vi "Get VIRef from ClassItem.vi"(8 "error in (no error)":errorcluster, 10 "Item Name":string, 11 "LVClassLibrary in":refnum<vi>) -> (0 "error out":errorcluster, 1 "Found ?":bool, 2 "VIref out":refnum<vi>, 3 "LVClassLibrary out":refnum<vi>)   [LabVIEW 2019, in "gRPC Scripting Tools.lvlib"]
uses:
  gRPC Scripting Tools.lvlib
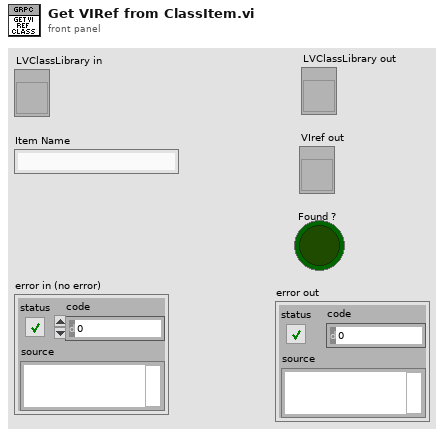
[diagram p1: front panel]
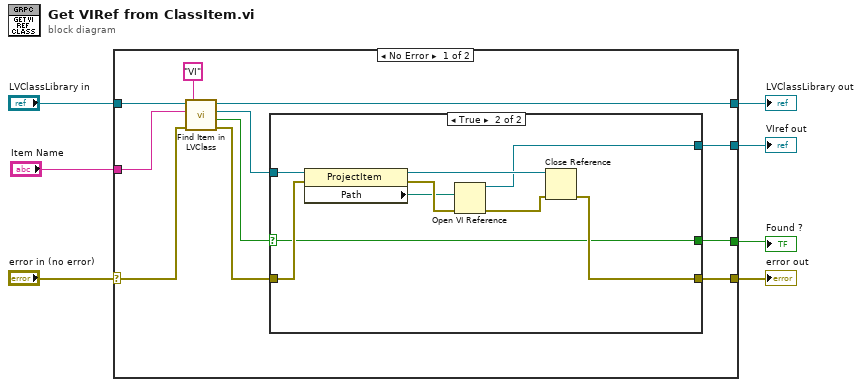
[diagram p0: block diagram]
diagram:
  n1 = case shown="No Error" "error in (no error)" {
    selector: "error in (no error)" -> [w11 w30]
    tunnel: "LVClassLibrary in" -> [w16 w31]
    tunnel: "Item Name" -> [w14 _]
    tunnel: [w13 w31] -> w5
    tunnel: [w12 w30] -> w4
    tunnel: [w9 _] -> w2
    tunnel: [w8 _] -> w1
    frame No Error {
      n2 = call "Find Item in LVClass.vi"("Item Type"="VI", "error in (no error)"=w11, "Item Name"=w14, "Class Item in"=w16) -> ("error out"=w18:errorcluster, "Found?"=w10:bool, "Project Item (Class Item)"=w17:refnum<vi>, "Class Item out"=w13:refnum<vi>)  [unwired: 4 in]
      n3 = case shown="True" w10 {
        selector: w10 -> [w19 w23]
        tunnel: w18 -> [w20 w28]
        tunnel: w17 -> [_ w27]
        tunnel: [w20 w24] -> w12
        tunnel: [w19 w23] -> w9
        tunnel: [_ w21] -> w8
        frame False {
        }
        frame True {
          n4 = property class="ProjectItem"(reference=w27, error in=w28) -> (reference out=w25:refnum<vi>, error out=w29:errorcluster, "Path"=w26:path)
          n5 = Open VI Reference(vi path=w26, error in (no error)=w29) -> (vi reference=w21:refnum<vi>, error out=w22:errorcluster)  [unwired: 4 in]
          n6 = Close Reference(reference=w25, error in (no error)=w22) -> (error out=w24:errorcluster)
        }
      }
    }
    frame Error {
    }
  }
  "LVClassLibrary out" <- w5
  "error out" <- w4
  "Found ?" <- w2
  "VIref out" <- w1
